vi "Downsample v2.vi"(10 "Divide by":i32, 11 "Waveform in":waveform(dbl)) -> (3 "Waveform out":waveform(dbl))   [LabVIEW 2017]
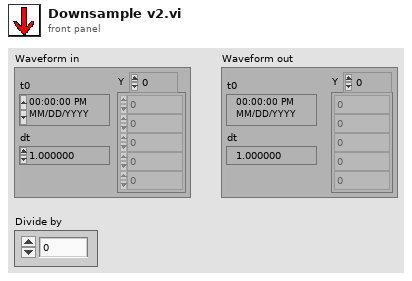
[diagram p1: front panel]
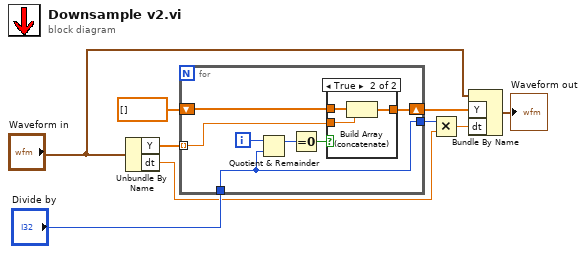
[diagram p0: block diagram]
diagram:
  n1 = Unbundle By Name("Waveform in") -> ("Y"=w2:dbl[], "dt"=w6:dbl)
  n2 = for {
    tunnel: w2 -> [w14] mode=indexing
    shift-right: [w16] -> w4
    shift-left: dbl[] [] ("Y") -> [w15]
    tunnel: [w10] -> w7
    tunnel: "Divide by" -> [w10]
    i -> [w12]
    n3 = Quotient & Remainder(x=w12, y=w10) -> (x-y*floor(x/y)=w13:i32)  [unwired: 1 out]
    n4 = Equal To 0?(x=w13) -> (x = 0?=w11:bool)
    n5 = case shown="True" w11 {
      tunnel: [w17 w20] -> w16
      tunnel: w15 -> [w17 w19]
      tunnel: w14 -> [_ w18]
      frame False {
      }
      frame True {
        n6 = Build Array (concatenate)(w19, w18) -> (w20:dbl[])
      }
    }
  }
  n7 = Multiply(x=w7, y=w6) -> (x*y=w5:dbl)
  n8 = Bundle By Name(cluster="Waveform in", "Y"=w4, "dt"=w5) -> (→"Waveform out":waveform(dbl))
